vi "Log Error.vi"(10 "error in":errorcluster, 11 "Console Log in":refnum<class "Console Log.lvclass">) -> (2 "error out":errorcluster, 3 "Console Log out":refnum<class "Console Log.lvclass">)   [LabVIEW 2017, in "Console Log.lvclass"]
uses:
  Console Log.lvclass
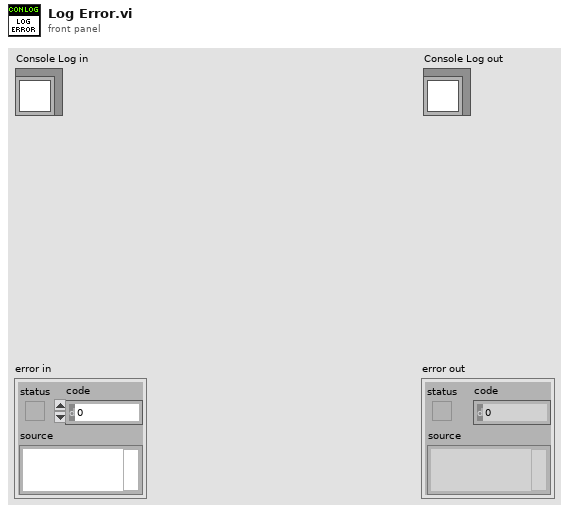
[diagram p1: front panel]
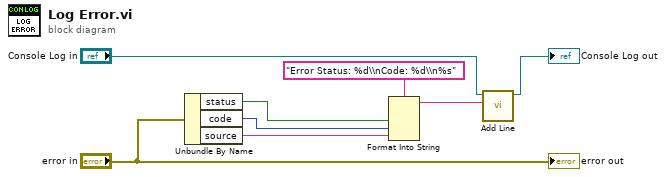
[diagram p0: block diagram]
diagram:
  n1 = Unbundle By Name("error in") -> ("status"=w6:bool, "code"=w5:i32, "source"=w4:string)
  n2 = Format Into String(format string="Error Status: %d\\nCode: %d\\n%s", w6, w5, w4) -> (resulting string=w2:string)  [unwired: 2 in, 1 out]
  n3 = call "Add Line.vi"("String"=w2, "Console Log in"="Console Log in") -> ("Console Log out"=→"Console Log out":refnum<class "Console Log.lvclass">)  [unwired: 8 in, 1 out]
  "error out" <- "error in"
